vi "Smart IO Get Counter.vi"(8 "error in (no error)":errorcluster, 11 "deviceIndex":i32) -> (0 "error out":errorcluster, 2 "count out":i32)   [LabVIEW 2026, in "MrcLib.lvlib"]
doc: "Return the current count of a device channel configured for up or down counting."
uses:
  MrcLib.lvlib
  Types/MRC Smart IO Mode.ctl
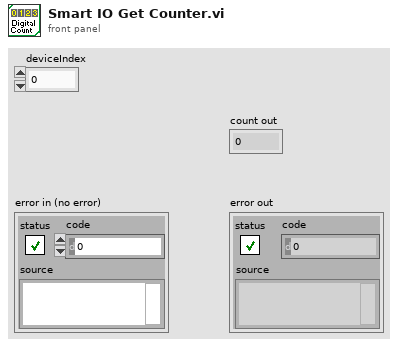
[diagram p1: front panel]
types:
  T1 = typedef "MRC Smart IO Mode.ctl" = i32
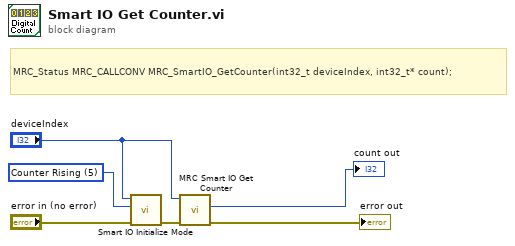
[diagram p0: block diagram]
diagram:
  w1 = T1 5 items=["Digital Input"=0, "Digital Output"=1, "Analog Input"=2, "PWM Input"=3, "PWM Output"=4, "Counter Rising"=5, "Counter Falling"=6, "Addressable LEDs"=13] ("mode")
  # "MRC_Status MRC_CALLCONV MRC_SmartIO_GetCounter(int32_t deviceIndex, int32_t* count);"
  n1 = call "Smart IO Initialize Mode.vi"("error in (no error)"="error in (no error)", "mode"=w1, "deviceIndex"="deviceIndex") -> ("error out"=w3:errorcluster)  [unwired: 8 in]
  n2 = call "MRC Smart IO Get Counter.vi"("error in (no error)"=w3, "deviceIndex"="deviceIndex") -> ("error out"=→"error out":errorcluster, "count out"=→"count out":i32)  [unwired: 8 in]
